vi "Read Y.vi"(8 "error in (no error)":errorcluster, 11 "Mouse Macro in":refnum<class "Mouse Macro.lvclass">) -> (0 "error out":errorcluster, 2 "Y":i32, 3 "Mouse Macro out":refnum<class "Mouse Macro.lvclass">)   [LabVIEW 2020, in "MacroAssert.lvlib" / "Mouse Macro.lvclass"]
uses:
  Mouse Macro.lvclass
  Mouse Macro.lvclass/Mouse Macro.ctl
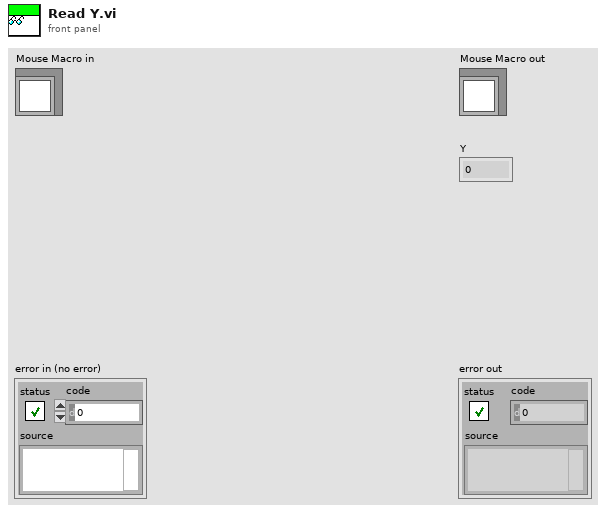
[diagram p1: front panel]
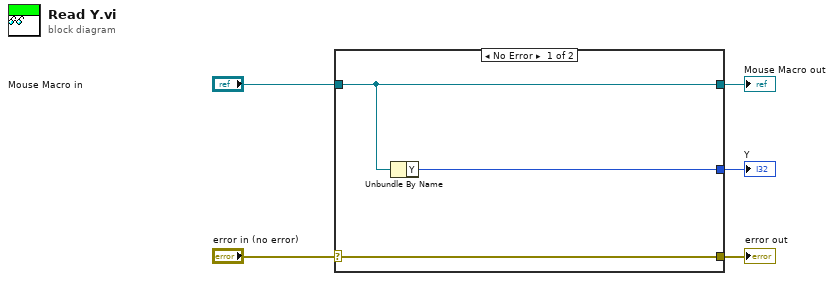
[diagram p0: block diagram]
diagram:
  n1 = case shown="No Error" "error in (no error)" {
    selector: "error in (no error)" -> [w8 w9]
    tunnel: [w8 w9] -> w4
    tunnel: [w7 w10] -> w2
    tunnel: "Mouse Macro in" -> [w7 w10]
    tunnel: [w6 _] -> w1
    frame No Error {
      n2 = Unbundle By Name(w7) -> ("Y"=w6:i32)
    }
    frame Error {
    }
  }
  "error out" <- w4
  "Mouse Macro out" <- w2
  "Y" <- w1
